vi "replace_array_row_by_element.vi"(8 "error_in":errorcluster, 9 "index (row)":i32, 10 "Array in":sgl[][](array[numeric]), 11 "element":dbl) -> (0 "error_out":errorcluster, 3 "Array out":sgl[][](array[numeric]))   [LabVIEW 2017]
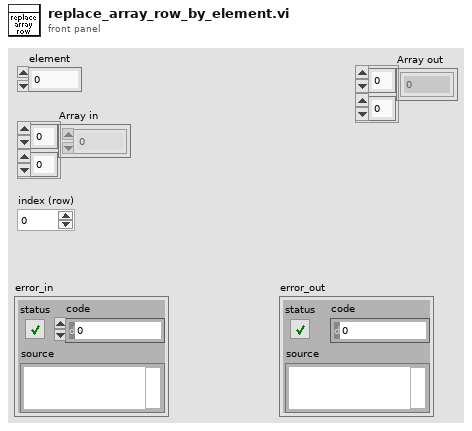
[diagram p1: front panel]
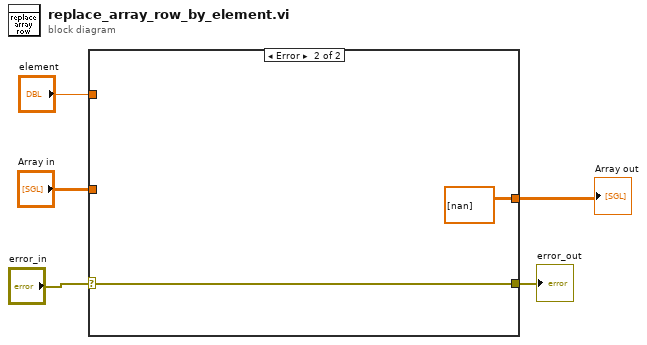
[diagram p0: block diagram]
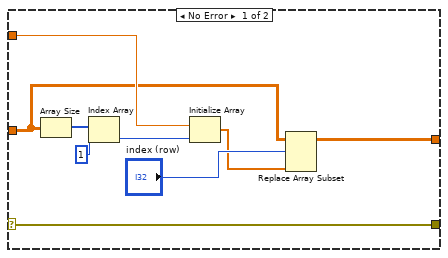
[diagram p2: hidden frame]
diagram:
  n1 = case shown="Error" "error_in" {
    selector: "error_in" -> [w6 w16]
    tunnel: "element" -> [w14 _]
    tunnel: [w13 sgl[][] [[nan]] ("Array in")] -> w4
    tunnel: "Array in" -> [w10 _]
    tunnel: [w6 w16] -> w2
    frame No Error {
      n2 = Array Size(array=w10) -> (size(s)=w7:i32[])
      n3 = Index Array(array=w7, index=1) -> (element=w9:i32)
      n4 = Initialize Array(w14, w9) -> (w11:dbl[])
      n5 = Replace Array Subset(array=w10, new element=w11, index (row)="index (row)") -> (w13:sgl[][])  [unwired: 1 in]
    }
    frame Error {
    }
  }
  "Array out" <- w4
  "error_out" <- w2
